vi "Flywheel Control.vi"(0 "I in":dbl=-0.027, 1 "P in":dbl=20.0 step=0.1, 5 "D in":dbl=-0.008, 7 "F":dbl, 9 "I Zone in":dbl, 11 "CAN Talon SRX Ref":T2={"DeviceStatus"={"status"=FALSE, "code"=0, "source"=""}, "Type"=enum."CAN", "PWM"={"PWM Channel"=enum."PWM 1", "DeadBand"={"Name"="", "maxPositivePwm"=0, "minPositivePwm"=0, "centerPwm"=0, "maxNegativePwm"=0, "minNegativePwm"=0, "angularRange"=0}}, "CAN"={"Device Number"=1, "SetOutput VI Ref"=variant(refnum<vi> refnum), "GetOutput VI Ref"=variant(refnum<vi> refnum), "Enable VI Ref"=variant(refnum<vi> refnum), "Disable VI Ref"=variant(refnum<vi> refnum), "Data"=variant(cluster{"Control Mode":enum8{"Percent VBus", "Speed", "Position", "Slave", "Unchanged / Invalid", "Voltage Compensation", "Current", "Motion Profile", "Motion Magic"}, "Encoder Initial Position":dbl, "MaxVout":dbl} {"Control Mode"=enum."Speed", "Encoder Initial Position"=0.0, "MaxVout"=12.0})}, "Invert"=FALSE}, 12 "Ramp Rate in":dbl) -> (3 "Speed Closed Loop Plots":T6(graph)={"Sensor Velocity"=0.0, "Encoder Velocity"=0.0, "Encoder Position"=-479974.0}, 6 "Motor output Plot 2":cluster{"Applied Throttle":dbl}(graph), 8 "SensorRPM Velocity RPM 2":dbl, 10 "SensorPosRotations":dbl=17141.928571428572, 14 "Applied Output 2":dbl)   [LabVIEW 2016]
uses:
  <vilib>/Rock Robotics/WPI/MotorControl/WPI_MotorControlDeviceRef.ctl
  <vilib>/Rock Robotics/WPI/MotorControl/WPI_MotorControlType.ctl
  <vilib>/Rock Robotics/SystemInterfaces/DIO/FPGA_DIOPWMChannel.ctl
  <vilib>/Rock Robotics/WPI/PWM/WPI_PWMDeadband.ctl
  <vilib>/Rock Robotics/WPI/ThirdParty/CanMotor/TalonSRX/WPI_CANTalonSRX_GlobalStatus.ctl
panel:
  in  "P in 2":dbl=9.0 step=0.1
  in  "D in 2":dbl
  in  "I in 2":dbl
  out "Talon SRX Status":T1={"Applied Throttle"=0.0, "Module Enabled"=FALSE, "CAN Error"={"status"=FALSE, "code"=0, "source"=""}, "Closed Loop Error"=33.0, "Forward Limit Switch Closed"=FALSE, "Reverse Limit Switch Closed"=FALSE, "Sensor Position"=17141.928571428572, "Sensor Velocity"=0.0, "Current"=0.125, "Sticky Fault - Over Temp"=FALSE, "Sticky Fault - Under Voltage"=TRUE, "Sticky Fault - Forward Limit"=FALSE, "Sticky Fault - Reverse Limit"=FALSE, "Sticky Fault - Forward Soft Limit"=FALSE, "Sticky Fault - Reverse Soft Limit"=FALSE, "Brake is Enabled"=FALSE, "Encoder Position"=-479974.0, "Encoder Velocity"=0.0, "Encoder Index Count"=0.0, "Encoder A Pin State"=FALSE, "Encoder B Pin State"=TRUE, "Encoder Index Pin State"=TRUE, "Analog In"=99.0, "Analog In Velocity"=0.0, "Temperature (C)"=24.19354838709677, "Battery Voltage"=12.4, "Control 5 Is Supported"=TRUE, "Current Profile Slot Select"=0.0, "Pos Div 8"=FALSE, "Vel Div 4"=FALSE, "Pulse Width Position"=0, "Pulse Width Velocity"=0, "Pulse Width Rise To Rise (us)"=0, "Pulse Width Rise To Fall (us)"=0, "Mot Prof Active Is Under Run"=FALSE, "Mot Prof Active Has Under Run"=FALSE, "Mot Prof Active Is Last"=FALSE, "Mot Prof Active Velocity Only"=FALSE, "Mot Prof Active Is Valid"=FALSE, "Mot Prof Buffer Is Full"=FALSE, "Mot Prof Active Profile Slot Select"=0, "Mot Prof NextID"=0, "Mot Prof Count"=0, "Mot Prof Active Velocity"=0.0, "Mot Prof Active Position"=0.0, "Mot Prof Output Enable"=0, "UsageFrame"=5, "Motion Magic Active Trajectory"={"Velocity"=0.0, "Position"=0.0}}
  out "Encoder A Pin State":bool
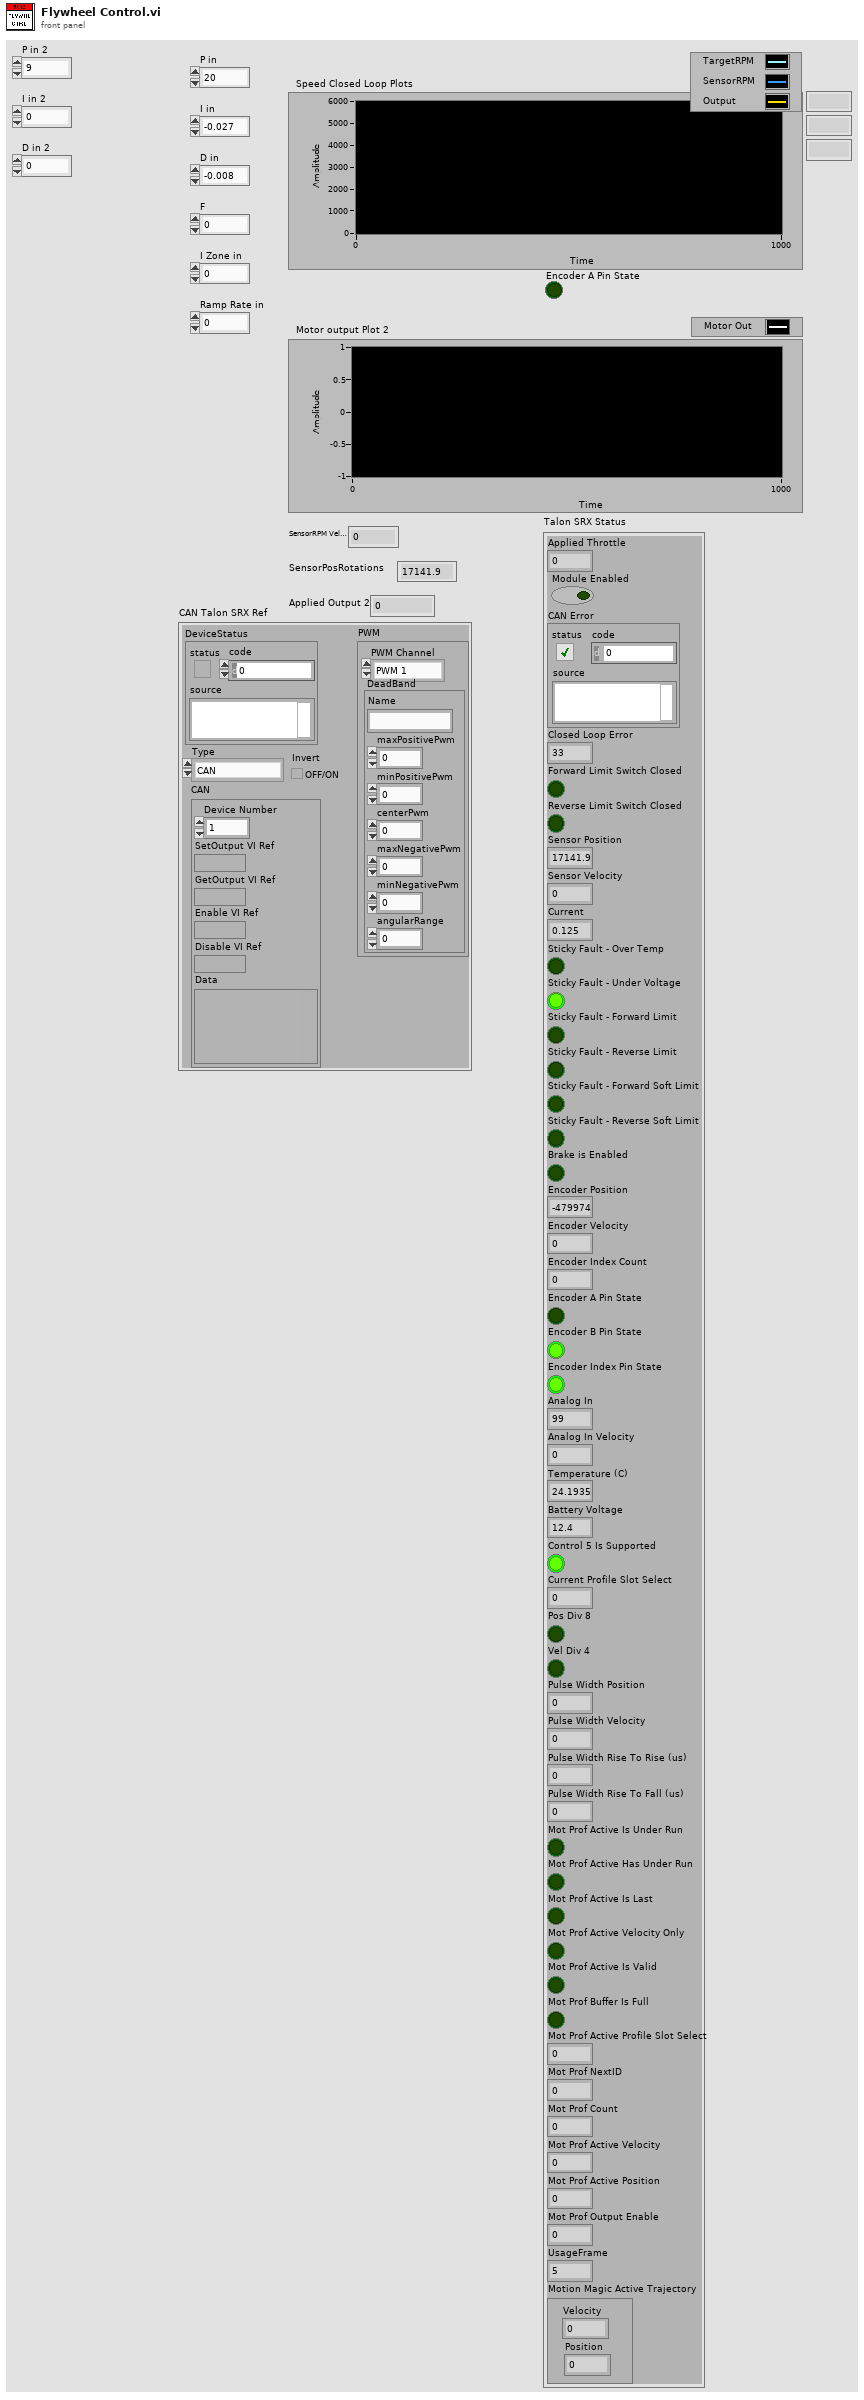
[diagram p1: front panel]
types:
  T1 = typedef "WPI_CANTalonSRX_GlobalStatus.ctl" = cluster{"Applied Throttle":dbl, "Module Enabled":bool, "CAN Error":errorcluster, "Closed Loop Error":dbl, "Forward Limit Switch Closed":bool, "Reverse Limit Switch Closed":bool, "Sensor Position":dbl, "Sensor Velocity":dbl, "Current":dbl, "Sticky Fault - Over Temp":bool, "Sticky Fault - Under Voltage":bool, "Sticky Fault - Forward Limit":bool, "Sticky Fault - Reverse Limit":bool, "Sticky Fault - Forward Soft Limit":bool, "Sticky Fault - Reverse Soft Limit":bool, "Brake is Enabled":bool, "Encoder Position":dbl, "Encoder Velocity":dbl, "Encoder Index Count":dbl, "Encoder A Pin State":bool, "Encoder B Pin State":bool, "Encoder Index Pin State":bool, "Analog In":dbl, "Analog In Velocity":dbl, "Temperature (C)":dbl, "Battery Voltage":dbl, "Control 5 Is Supported":bool, "Current Profile Slot Select":dbl, "Pos Div 8":bool, "Vel Div 4":bool, "Pulse Width Position":i32, "Pulse Width Velocity":i32, "Pulse Width Rise To Rise (us)":i32, "Pulse Width Rise To Fall (us)":i32, "Mot Prof Active Is Under Run":bool, "Mot Prof Active Has Under Run":bool, "Mot Prof Active Is Last":bool, "Mot Prof Active Velocity Only":bool, "Mot Prof Active Is Valid":bool, "Mot Prof Buffer Is Full":bool, "Mot Prof Active Profile Slot Select":i32, "Mot Prof NextID":i32, "Mot Prof Count":i32, "Mot Prof Active Velocity":dbl, "Mot Prof Active Position":dbl, "Mot Prof Output Enable":i32, "UsageFrame":u32, "Motion Magic Active Trajectory":cluster{"Velocity":dbl, "Position":dbl}}
  T2 = typedef "WPI_MotorControlDeviceRef.ctl" = cluster{"DeviceStatus":errorcluster, "Type":T3, "PWM":cluster{"PWM Channel":T4, "DeadBand":T5}, "CAN":cluster{"Device Number":u8, "SetOutput VI Ref":variant, "GetOutput VI Ref":variant, "Enable VI Ref":variant, "Disable VI Ref":variant, "Data":variant}, "Invert":bool}
  T3 = typedef "WPI_MotorControlType.ctl" = enum16{"PWM", "CAN"}
  T4 = typedef "FPGA_DIOPWMChannel.ctl" = enum8{"PWM 0", "PWM 1", "PWM 2", "PWM 3", "PWM 4", "PWM 5", "PWM 6", "PWM 7", "PWM 8", "PWM 9", "PWM MXP 0", "PWM MXP 1", "PWM MXP 2", "PWM MXP 3", "PWM MXP 4", "PWM MXP 5", "PWM MXP 6", "PWM MXP 7", "PWM MXP 8", "PWM MXP 9", "Invalid"}
  T5 = typedef "WPI_PWMDeadband.ctl" = cluster{"Name":string, "maxPositivePwm":i32, "minPositivePwm":i32, "centerPwm":i32, "maxNegativePwm":i32, "minNegativePwm":i32, "angularRange":u16}
  T6 = cluster{"Sensor Velocity":dbl, "Encoder Velocity":dbl, "Encoder Position":dbl}
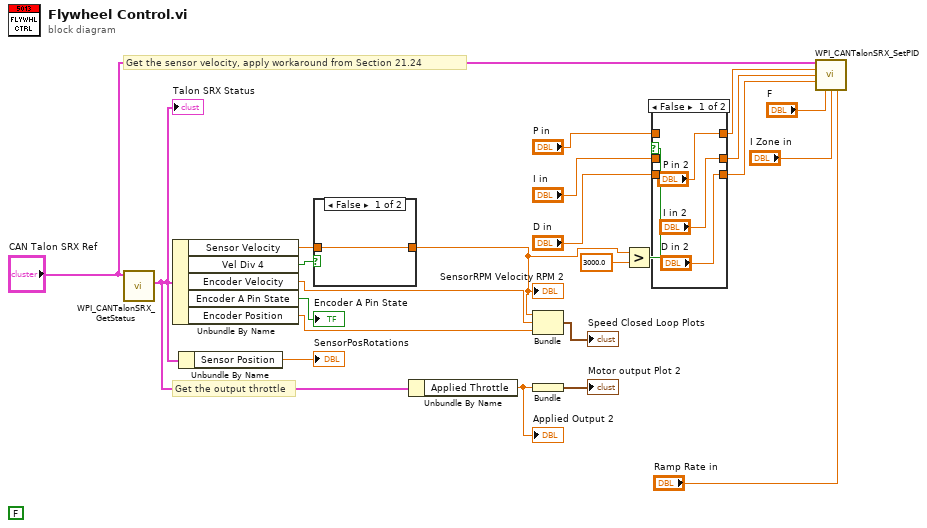
[diagram p0: block diagram]
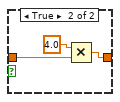
[diagram p3: hidden frame]
diagram:
  (unwired) FALSE
  # "Get the output throttle"
  # "Get the sensor velocity, apply workaround from Section 21.24"
  n1 = call <vilib>:"WPI_CANTalonSRX_GetStatus.vi"("CAN Talon SRX Ref"="CAN Talon SRX Ref") -> ("Talon SRX Status"=w19:T1)  [unwired: 8 in, 2 out]
  "Talon SRX Status" <- w19
  n2 = Unbundle By Name(w19) -> ("Sensor Velocity"=w10:dbl, "Vel Div 4"=w20:bool, "Encoder Velocity"=w14:dbl, "Encoder A Pin State"=→"Encoder A Pin State":bool, "Encoder Position"=w12:dbl)
  n3 = Unbundle By Name(w19) -> ("Sensor Position"=→"SensorPosRotations":dbl)
  n4 = case shown="False" w20 {
    tunnel: [w24 w26] -> w9
    tunnel: w10 -> [w24 w25]
    frame False {
    }
    frame True {
      n5 = Multiply(x=4.0, y=w25) -> (x*y=w26:dbl)
    }
  }
  "SensorRPM Velocity RPM 2" <- w9
  n6 = Unbundle By Name(w19) -> ("Applied Throttle"=w16:dbl)
  "Applied Output 2" <- w16
  n7 = Bundle("Sensor Velocity"=w9, "Encoder Velocity"=w14, "Encoder Position"=w12) -> (→"Speed Closed Loop Plots":T6)  [unwired: 1 in]
  n8 = Bundle("Applied Throttle"=w16) -> (→"Motor output Plot 2":cluster{"Applied Throttle":dbl})  [unwired: 1 in]
  n9 = Greater?(x=w9, y=3000.0) -> (0:w7:bool)
  n10 = case shown="False" w7 {
    tunnel: "P in" -> [_ w33]
    tunnel: "I in" -> [_ w32]
    tunnel: "D in" -> [_ w31]
    tunnel: ["P in 2" w33] -> w3
    tunnel: ["I in 2" w32] -> w2
    tunnel: ["D in 2" w31] -> w1
    frame False {
    }
    frame True {
    }
  }
  n11 = call <vilib>:"WPI_CANTalonSRX_SetPID.vi"("CAN Talon SRX Ref"="CAN Talon SRX Ref", "P"=w3, "I"=w2, "D"=w1, "F"="F", "I Zone"="I Zone in", "Ramp Rate"="Ramp Rate in") -> ()  [unwired: 7 in, 2 out]
